vi "enumerateStaticDependencies.vi"(8 "error in (no error)":errorcluster, 11 "Maui 2.0":refnum<class "Maui 2.0.lvclass">) -> (0 "error out":errorcluster, 2 "Static Dependencies":refnum<class "Dependency.lvclass">[](array[class]), 3 "Maui 2.0 out":refnum<class "Maui 2.0.lvclass">)   [LabVIEW 2020, in "Maui 2.0.lvclass"]
doc: "JKI State Machine Objects (SMO) 1.3.0.56\nJKI - JKI\nCopyright (c) 2017, JKI"
uses:
  Maui 2.0.lvclass
  <vilib>/JKI/JKI SMO/SMO/SMO.lvclass
  <vilib>/JKI/JKI SMO/Dependency/Dependency.lvclass
  Lifeguard/Lifeguard.lvclass
  C:/Program Files (x86)/National Instruments/LabVIEW 2020/vi.lib/JKI/JKI SMO/SMO/SMO.lvclass
  C:/Users/Albro/Documents/GitHub/MAUI-Engine/lvsrc/Maui 2.0/Lifeguard/Lifeguard.lvclass
panel:
  # "For instructions on how to use the JKI State Machine Objects, examples and video tutorials, visit:\nhttp://jki.net/state-machine-objects/\n\nJKI State Machine Objects™\nhttp://jki.net/state-machine-objects/\nCopyright (C) 2005-2015, JKI <info@jki.net>\nALL RIGHTS RESERVED"
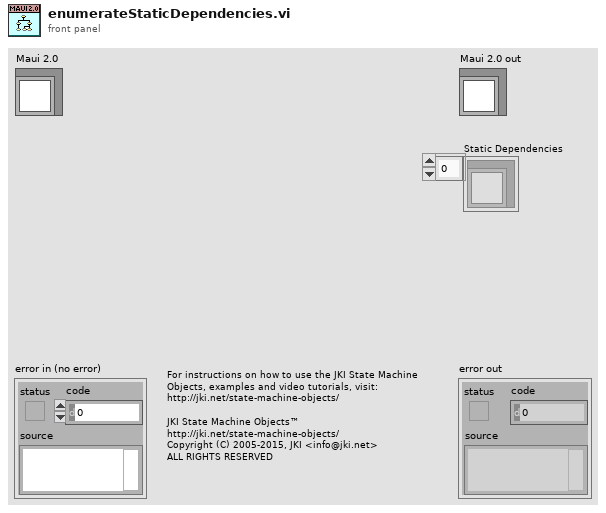
[diagram p1: front panel]
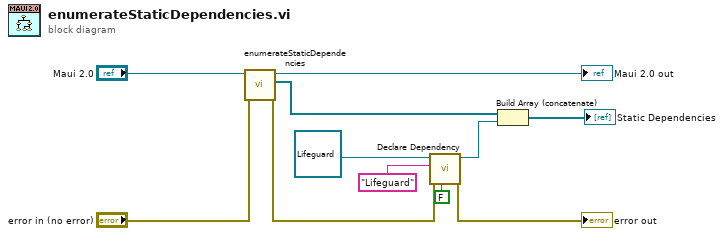
[diagram p0: block diagram]
diagram:
  n1 = call-parent "enumerateStaticDependencies.vi"("error in (no error)"="error in (no error)", "SMO"="Maui 2.0") -> ("error out"=w2:errorcluster, "Static Dependencies"=w4:refnum<class "Dependency.lvclass">[], "SMO out"=→"Maui 2.0 out":refnum<class "Maui 2.0.lvclass">)  [unwired: 7 in]
  n2 = call <vilib>:"Declare Dependency.vi"("Shared Resource (F)"=FALSE, "error in (no error)"=w2, "Name"="Lifeguard", "Type"=refnum<class "Lifeguard.lvclass"> refnum ("Lifeguard.lvclass")) -> ("error out"=→"error out":errorcluster, "Dependency out"=w5:refnum<class "Dependency.lvclass">)  [unwired: 6 in]
  n3 = Build Array (concatenate)(w4, w5) -> (→"Static Dependencies":refnum<class "Dependency.lvclass">[])
